vi "圆整到2的N次方.vi"(4 "Num":u32) -> (1 "2^N":u32)   [LabVIEW 2012]
doc: "功能：\n\n把给定的整数圆整到2的N次方。\n\n由于计算机内部是以字节为单位存储数据的，因此对于分配内存操作，分配为2的N次方大小对于提高运算性能是非常有益的。比如128、1024等等。\n\nLabVIEW的数据处理函数默认的就是128个采样点。\n\ncsxcs_366创建"
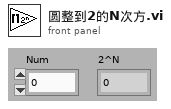
[diagram p1: front panel]
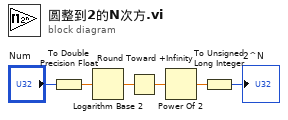
[diagram p0: block diagram]
diagram:
  n1 = To Double Precision Float(number="Num") -> (double precision float=w1:dbl)
  n2 = Logarithm Base 2(1:w1) -> (0:w6:dbl)
  n3 = Round Toward +Infinity(x=w6) -> (ceil(x): smallest int >= x=w5:dbl)
  n4 = Power Of 2(x=w5) -> (2^x=w3:dbl)
  n5 = To Unsigned Long Integer(number=w3) -> (unsigned 32bit integer=→"2^N":u32)
